vi "Blackman Window (CDB).vi"(0 "X":cdb[](array[numeric])) -> (1 "Windowed X":cdb[](array[numeric]), 2 "error":i32)   [LabVIEW 2017, in "NI_AALPro.lvlib"]
doc: "Applies a Blackman window to the input signal <B>X</B>. Wire data to the <B>X</B> input to determine the polymorphic instance to use or manually select the instance."
uses:
  NI_AALPro.lvlib
panel:
  # "Blackman Window"
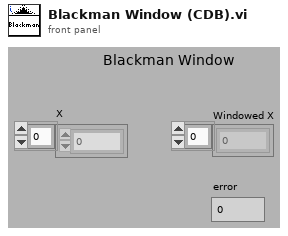
[diagram p1: front panel]
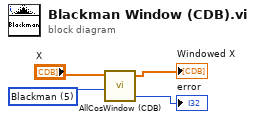
[diagram p0: block diagram]
diagram:
  w3 = u16 5 items=["None "=0, "Hanning"=1, "Hamming"=2, "Blackman-Harris"=3, "Exact Blackman"=4, "Blackman"=5, "Flat Top"=6, "4 Term B-Harris "=7, "7 Term B-Harris"=8, "Low Sidelobe"=9, "Blackman Nuttall"=14] ("window")
  n1 = call "AllCosWindow (CDB).vi"("window"=w3, "X"="X") -> ("error"=→"error":i32, "Windowed X"=→"Windowed X":cdb[])  [unwired: 3 in]
